vi "Close.vi"(8 "error in (no error)":errorcluster, 11 "Data":variant) -> (0 "error out":errorcluster)   [LabVIEW 2021, in "EOL Controller.lvlib"]
uses:
  EOL Controller.lvlib
  Private Controls/Module Action.ctl
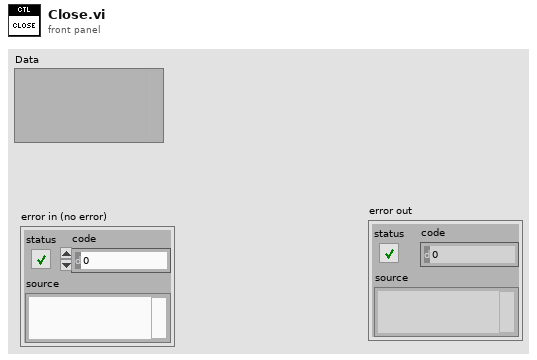
[diagram p1: front panel]
types:
  T1 = typedef "EOL Controller.lvlib/Module Action.ctl" = enum16{"Init", "Error", "Close", "PreUUT", "Test Execution", "PostUUT"}
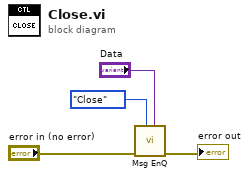
[diagram p0: block diagram]
diagram:
  n1 = call "Msg EnQ.vi"("Data"="Data", "Module Action"=Module_Action."Close", "error in (no error)"="error in (no error)") -> ("error out"=→"error out":errorcluster)  [unwired: 8 in]
